vi "Build.vi"(8 "error in":errorcluster) -> (0 "error out":errorcluster)   [LabVIEW 2020, in "CICD.lvlib"]
doc: "Build the EXE using the build spec in the .lvproj file.\nThe function accepts the following paramerters:\n -ProjectPath $ProjectPath Path to the LabVIEW project (.lvproj) that contains the build spec`\n -BuildSpecName Name of the build spec in the project `\n -DestinationDir Destination for the build output `\n -VersionString Version in the format v<Major>.<Minor>.<Patch>somestring `\n -EnableDebugging Enable debugging in the built executable, default is false `\n -WaitForDebugger Wait for the debugger to create a connection before launching the built app, default is false"
uses:
  CICD.lvlib
  <vilib>/Wiresmith Technology/G CLI/CLI Class/CLI.lvclass
  <vilib>/Wiresmith Technology/G CLI/Argument Parser/Option Set Class/Option Set.lvclass
  <vilib>/Wiresmith Technology/G CLI/Argument Parser/Option Class/Option Configuration.ctl
  <vilib>/Wiresmith Technology/G CLI/Argument Parser/Option Class/Option.lvclass
  <vilib>/Wiresmith Technology/G CLI/Argument Parser/Option Class/Argument Type.ctl
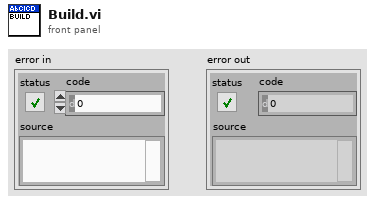
[diagram p1: front panel]
types:
  T1 = typedef "Option Parser.lvlib/Option.lvclass/Option Configuration.ctl" = cluster{"Option Type":T2, "Option Labels":string[], "Key":string, "Description":string, "Required":bool, "Default Value":string}
  T2 = typedef "Option Parser.lvlib/Option.lvclass/Argument Type.ctl" = enum16{"flag", "value"}
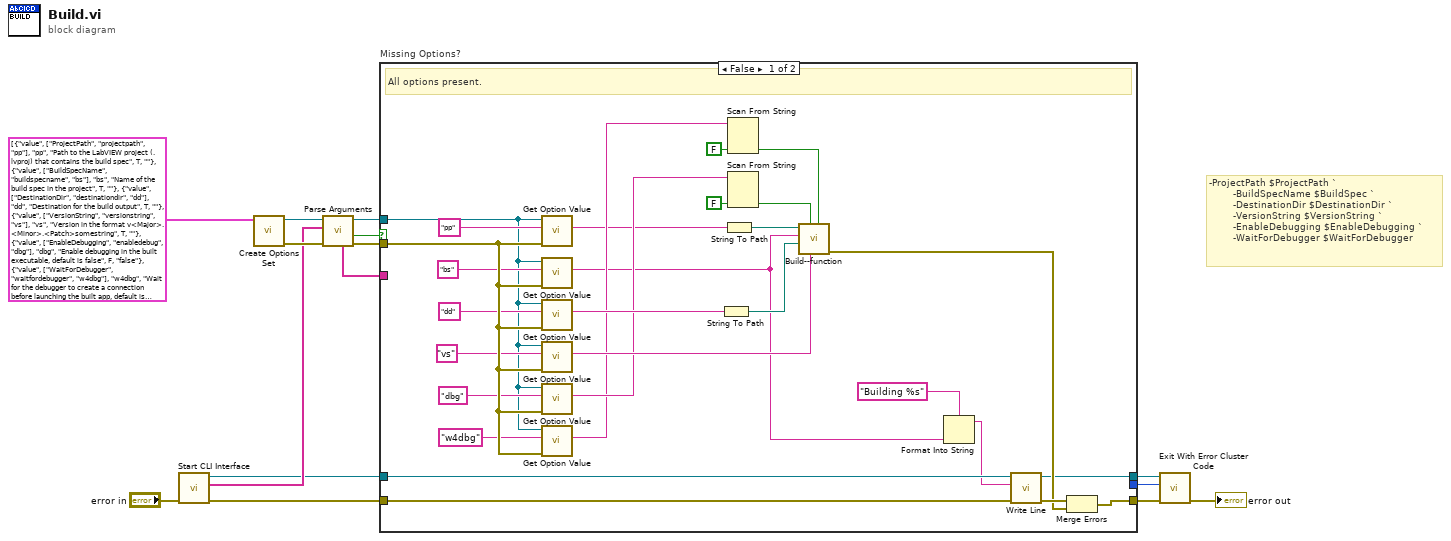
[diagram p0: block diagram]
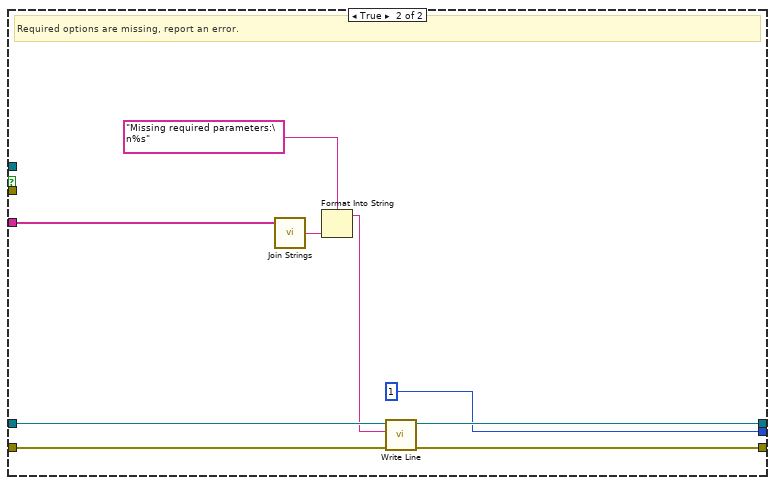
[diagram p2: hidden frame]
diagram:
  # "-ProjectPath $ProjectPath `\n        -BuildSpecName $BuildSpec `\n        -DestinationDir $DestinationDir `\n        -VersionString $VersionString `\n        -EnableDebugging $EnableDebugging `\n        -WaitForDebugger $WaitForDebugger"
  n1 = call <vilib>:"Start CLI Interface.vi"("error in (no error)"="error in") -> ("error out"=w12:errorcluster, "Custom Parameters"=w7:string[], "CLI out"=w4:refnum<class "CLI.lvclass">)  [unwired: 7 in, 1 out]
  n2 = call <vilib>:"Create Options Set.vi"("Options"=T1[] [{"Option Type"=enum."value", "Option Labels"=["ProjectPath", "projectpath", "pp"], "Key"="pp", "Description"="Path to the LabVIEW project (.lvproj) that contains the build spec", "Required"=TRUE, "Default Value"=""}, {"Option Type"=enum."value", "Option Labels"=["BuildSpecName", "buildspecname", "bs"], "Key"="bs", "Description"="Name of the build spec in the project", "Required"=TRUE, "Default Value"=""}, {"Option Type"=enum."value", "Option Labels"=["DestinationDir", "destinationdir", "dd"], "Key"="dd", "Description"="Destination for the build output", "Required"=TRUE, "Default Value"=""}, {"Option Type"=enum."value", "Option Labels"=["VersionString", "versionstring", "vs"], "Key"="vs", "Description"="Version in the format v<Major>.<Minor>.<Patch>somestring", "Required"=TRUE, "Default Value"=""}, {"Option Type"=enum."value", "Option Labels"=["EnableDebugging", "enabledebug", "dbg"], "Key"="dbg", "Description"="Enable debugging in the built executable, default is false", "Required"=FALSE, "Default Value"="false"}, {"Option Type"=enum."value", "Option Labels"=["WaitForDebugger", "waitfordebugger", "w4dbg"], "Key"="w4dbg", "Description"="Wait for the debugger to create a connection before launching the built app, default is false", "Required"=FALSE, "Default Value"="false"}]) -> ("error out"=w14:errorcluster, "Option Set out"=w9:refnum<class "Option Set.lvclass">)  [unwired: 9 in]
  n3 = call <vilib>:"Parse Arguments.vi"("error in (no error)"=w14, "Arguments"=w7, "Option Set in"=w9) -> ("error out"=w13:errorcluster, "Missing Options"=w6:bool, "Option Set out"=w1:refnum<class "Option Set.lvclass">, "Missing Option Keys"=w5:string[])  [unwired: 5 in]
  n4 = case "Missing Options?" shown="False" w6 {
    tunnel: w13 -> [w40 _]
    tunnel: w5 -> [_ w48]
    tunnel: w12 -> [w43 w52]
    tunnel: w4 -> [w38 w47]
    tunnel: [w41 w51] -> w11
    tunnel: [w37 w45] -> w3
    tunnel: [_ 1 ("No Error Code (0)")] -> w2
    tunnel: w1 -> [w30 _]
    frame False {
      # "All options present."
      n5 = call <vilib>:"Get Option Value.vi"("error in (no error)"=w40, "Option Key"="pp", "Option Set in"=w30) -> ("Value"=w19:string)  [unwired: 5 in, 3 out]
      n6 = call <vilib>:"Get Option Value.vi"("error in (no error)"=w40, "Option Key"="bs", "Option Set in"=w30) -> ("Value"=w17:string)  [unwired: 5 in, 3 out]
      n7 = call <vilib>:"Get Option Value.vi"("error in (no error)"=w40, "Option Key"="dd", "Option Set in"=w30) -> ("Value"=w28:string)  [unwired: 5 in, 3 out]
      n8 = call <vilib>:"Get Option Value.vi"("error in (no error)"=w40, "Option Key"="vs", "Option Set in"=w30) -> ("Value"=w26:string)  [unwired: 5 in, 3 out]
      n9 = call <vilib>:"Get Option Value.vi"("error in (no error)"=w40, "Option Key"="dbg", "Option Set in"=w30) -> ("Value"=w24:string)  [unwired: 5 in, 3 out]
      n10 = call <vilib>:"Get Option Value.vi"("error in (no error)"=w40, "Option Key"="w4dbg", "Option Set in"=w30) -> ("Value"=w21:string)  [unwired: 5 in, 3 out]
      n11 = String To Path(string=w28) -> (path=w27:path)
      n12 = String To Path(string=w19) -> (path=w29:path)
      n13 = Scan From String(input string=w21, default 1=FALSE) -> (output 1=w20:bool)  [unwired: 3 in, 3 out]
      n14 = Scan From String(input string=w24, default 1=FALSE) -> (output 1=w23:bool)  [unwired: 3 in, 3 out]
      n15 = call "Build--function.vi"("Wait for debugger on launch (false)"=w20, "VersionString"=w26, "Enable debugging (false)"=w23, "DestinationDir"=w27, "BuildSpec"=w17, "ProjectPath"=w29) -> ("error out"=w39:errorcluster)  [unwired: 4 in, 1 out]
      n16 = Format Into String(format string="Building %s", w17) -> (resulting string=w16:string)  [unwired: 2 in, 1 out]
      n17 = call <vilib>:"Write Line.vi"("error in (no error)"=w43, "Text to Write"=w16, "CLI in"=w38) -> ("error out"=w42:errorcluster, "CLI out"=w37:refnum<class "CLI.lvclass">)  [unwired: 7 in]
      n18 = Merge Errors(w42, w39) -> (w41:errorcluster)
    }
    frame True {
      # "Required options are missing, report an error."
      n19 = call <vilib>:"Join Strings.vi"("Strings In"=w48) -> ("String"=w49:string)  [unwired: 2 in]
      n20 = Format Into String(format string="Missing required parameters:\n%s" ("Text to Write"), w49) -> (resulting string=w46:string)  [unwired: 2 in, 1 out]
      n21 = call <vilib>:"Write Line.vi"("error in (no error)"=w52, "Text to Write"=w46, "CLI in"=w47) -> ("error out"=w51:errorcluster, "CLI out"=w45:refnum<class "CLI.lvclass">)  [unwired: 7 in]
    }
  }
  n22 = call <vilib>:"Exit With Error Cluster Code.vi"("error in (no error)"=w11, "No Error Code (0)"=w2, "CLI in"=w3) -> ("error out"=→"error out":errorcluster)  [unwired: 8 in]
